vi "HexString Boolean OR.vi"(0 "String":string, 7 "String 2":string, 11 "Error In":errorcluster) -> (4 "String_Out":string, 15 "Error Out":errorcluster)   [LabVIEW 2016]
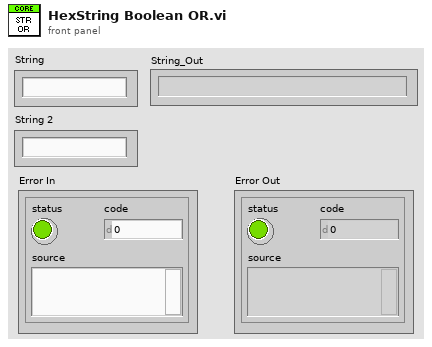
[diagram p1: front panel]
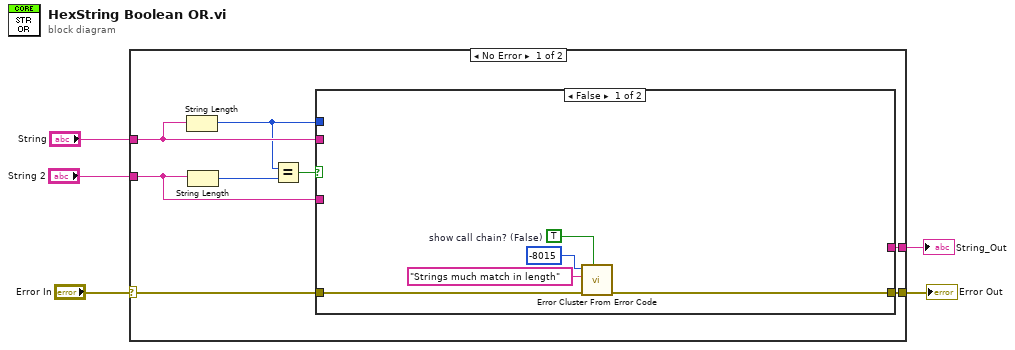
[diagram p0: block diagram]
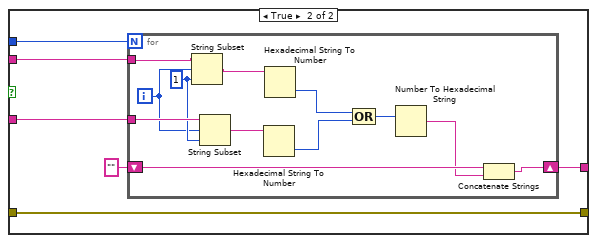
[diagram p2: hidden frame]
diagram:
  n1 = case shown="No Error" "Error In" {
    selector: "Error In" -> [w6 w37]
    tunnel: "String" -> [w13 _]
    tunnel: "String 2" -> [w10 _]
    tunnel: [w8 _] -> w3
    tunnel: [w7 w37] -> w1
    frame No Error {
      n2 = String Length(string=w13) -> (length=w11:i32)
      n3 = String Length(string=w10) -> (length=w12:i32)
      n4 = Equal?(x=w11, y=w12) -> (x = y?=w9:bool)
      n5 = case shown="False" w9 {
        tunnel: w13 -> [_ w24]
        tunnel: w11 -> [_ w23]
        tunnel: w10 -> [_ w22]
        tunnel: [_ w20] -> w8
        tunnel: [w17 w19] -> w7
        tunnel: w6 -> [w18 w19]
        frame False {
          w14 = TRUE  # show call chain? (False)
          n6 = call <vilib>:"Error Cluster From Error Code.vi"("show call chain? (False)"=w14, "error in (no error)"=w18, "error message (\"\")"="Strings much match in length" ("error message (\"\")"), "error code (0)"=-8015) -> ("error out"=w17:errorcluster)  [unwired: 5 in]
        }
        frame True {
          n7 = for {
            N: w23 -> [_]
            tunnel: w24 -> [w36]
            tunnel: w22 -> [w34]
            shift-right: [w27] -> w20
            shift-left: "" -> [w26]
            i -> [w32]
            w33 = 1 ("length (rest)")
            n8 = String Subset(string=w36, offset (0)=w32, length (rest)=w33) -> (substring=w35:string)
            n9 = String Subset(string=w34, offset (0)=w32, length (rest)=w33) -> (substring=w31:string)
            n10 = Hexadecimal String To Number(string=w31) -> (number=w29:u32)  [unwired: 2 in, 1 out]
            n11 = Hexadecimal String To Number(string=w35) -> (number=w30:u32)  [unwired: 2 in, 1 out]
            n12 = Compound Arithmetic op=OR(w30, w29) -> (w28:u32)
            n13 = Number To Hexadecimal String(2:w28) -> (0:w25:string)  [unwired: 1 in]
            n14 = Concatenate Strings(w26, w25) -> (w27:string)
          }
        }
      }
    }
    frame Error {
    }
  }
  "String_Out" <- w3
  "Error Out" <- w1
